vi "AP2_PDS_aquisition.vi"() -> ()   [LabVIEW 2023]
panel:
  in  "Frequency Doubling":bool
  out "RT PDS":cluster{dbl[], i32[]}(graph)
  in  "Cancel Scan Button":bool
  out "FPS":dbl
  in  "Frame timeout (ms)":u32
  in  "Number of buffers":u32
  in  "Region of interest":i32[](array[numeric])
  in  "Stop":bool
  in  "Aquistion Frame Number":i32
  in  "Lower Bound":dbl
  in  "Step Size":dbl
  in  "Upper bound":dbl
  in  "Scan button":bool
  # "AP-2 PDS Acquisition"
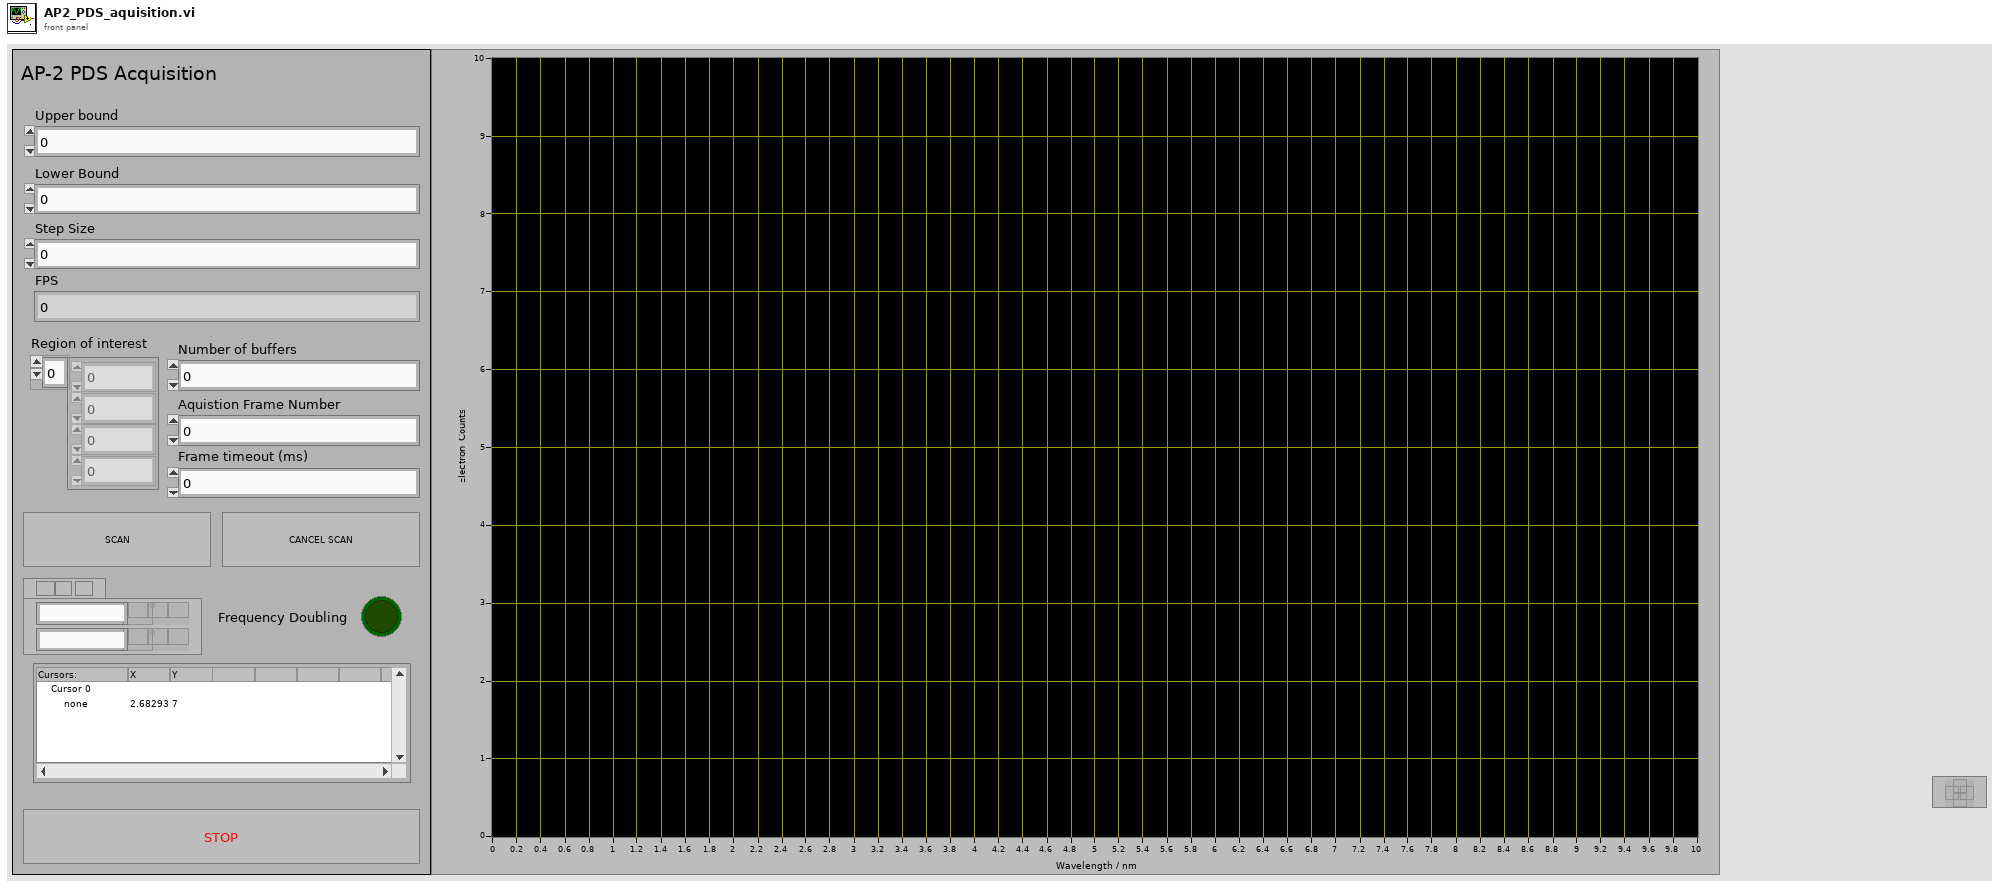
[diagram p1: front panel]
types:
  T1 = cluster{"Region of interest":i32[], "Number of buffers":u32, "Frame timeout (ms)":u32}
  T2 = cluster{"queue out":refnum<queue>, "error out":errorcluster}
  T3 = cluster{"Upper bound":dbl, "Step Size":dbl, "Lower Bound":dbl}
  T4 = cluster{"notifier out":refnum<notifier>, "error out":errorcluster}
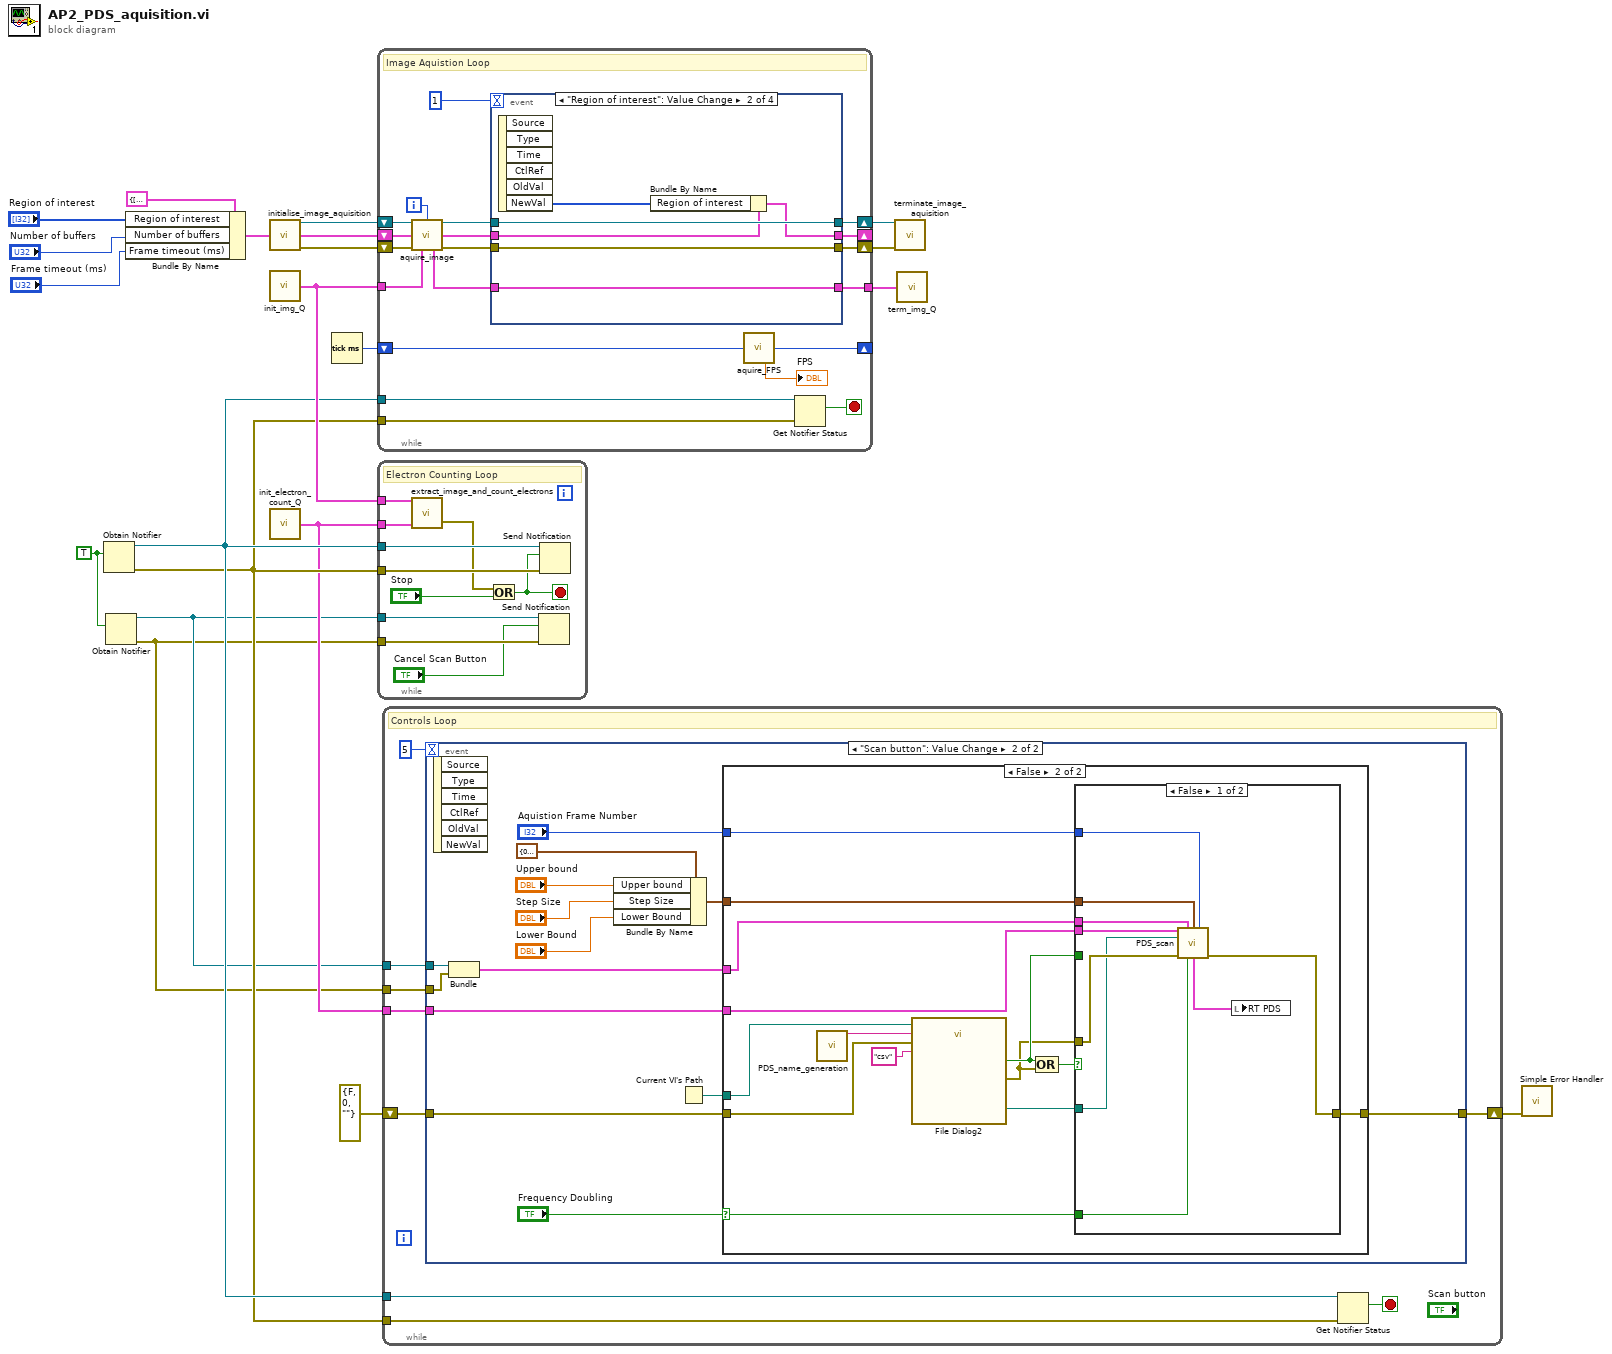
[diagram p0: block diagram]
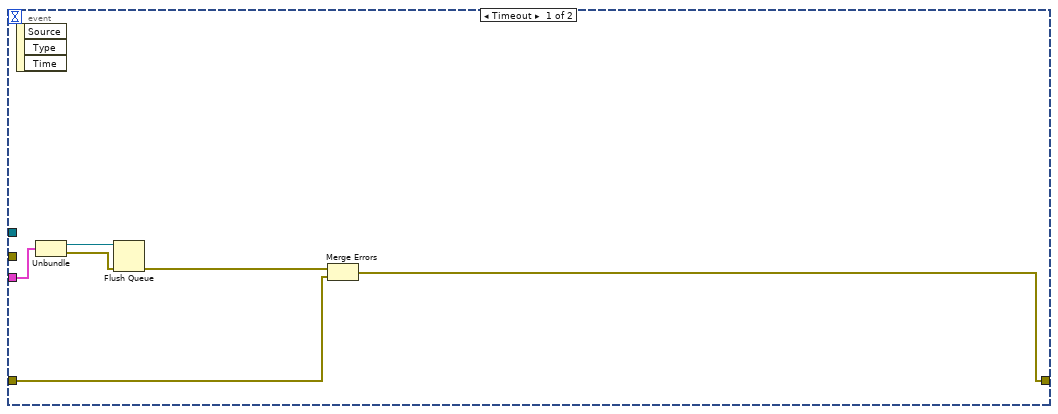
[diagram p2: hidden frame]
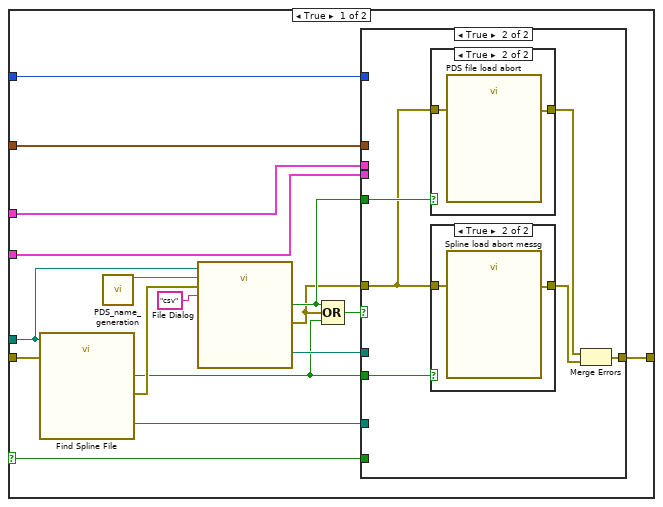
[diagram p3: hidden frame]
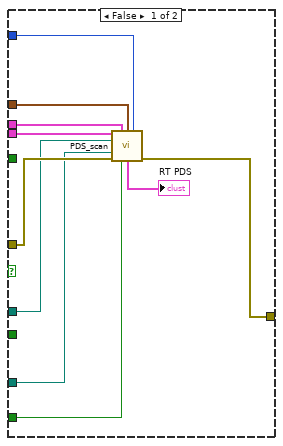
[diagram p4: hidden frame]
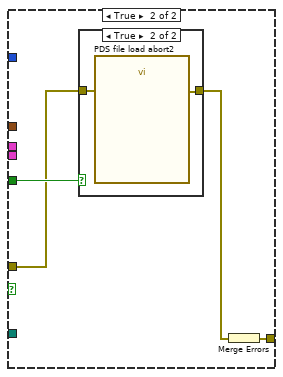
[diagram p7: hidden frame]
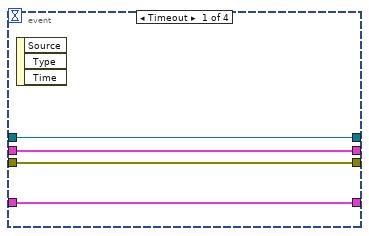
[diagram p9: hidden frame]
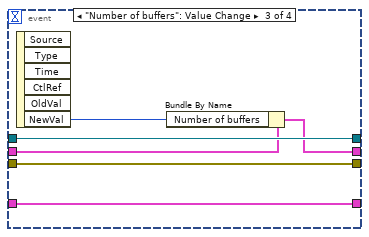
[diagram p10: hidden frame]
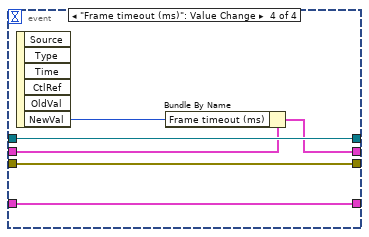
[diagram p11: hidden frame]
diagram:
  w3 = TRUE
  n1 = Obtain Notifier(notification data type=w3) -> (notifier out=w11:refnum<notifier>, error out=w7:errorcluster)  [unwired: 3 in, 1 out]
  n2 = Obtain Notifier(notification data type=w3) -> (notifier out=w2:refnum<notifier>, error out=w1:errorcluster)  [unwired: 3 in, 1 out]
  n3 = Bundle By Name(cluster=T1 {"Region of interest"=[], "Number of buffers"=0, "Frame timeout (ms)"=1000}, "Region of interest"="Region of interest", "Number of buffers"="Number of buffers", "Frame timeout (ms)"="Frame timeout (ms)") -> (w18:T1)
  n4 = call "initialise_image_aquisition.vi"("Imaging Variables In"=w18) -> ("IMAQ Session Out"=w21:refnum<k11>, "Imaging Variables Out"=w17:T1, "error out"=w20:errorcluster)  [unwired: 11 in, 1 out]
  n5 = call "init_img_Q.vi"() -> ("Image Q Out"=w12:T2)  [unwired: 15 in]
  n6 = call "init_electron_count_Q.vi"() -> ("Electron Count Q Out"=w4:T2)  [unwired: 15 in]
  n7 = Tick Count (ms)() -> (millisecond timer value=w13:u32)
  n8 = while {
    shift-right: [w40] -> w15
    shift-left: w21 -> [w37]
    shift-right: [w38] -> w14
    shift-left: w20 -> [w36]
    tunnel: w12 -> [w29]
    tunnel: [w28] -> w16
    shift-right: [w39] -> _
    shift-left: w17 -> [w32]
    shift-right: [w26] -> _
    shift-left: w13 -> [w27]
    tunnel: w11 -> [w25]
    tunnel: w7 -> [w24]
    i -> [w35]
    stop <- w23 stop-if-true
    # "Image Aquistion Loop"
    n9 = call "aquire_image.vi"("IMAQ Session In"=w37, "Buffer to extract"=w35, "Imaging Variables In"=w32, "error in (no error)"=w36, "Img Q Data In"=w29) -> ("IMAQ Session Out"=w34:refnum<k11>, "Imaging Variables Out"=w31:T1, "Img Q Data Out"=w30:T2, "error out"=w33:errorcluster)  [unwired: 7 in]
    n10 = event shown="[1] \"Region of interest\": Value Change" {
      selector: _ -> [_ _ _ _]
      dyn-events: _ -> [_ _ _ _]
      timeout: 1 -> [_ _ _ _]
      tunnel: w34 -> [w45 w51 w57 w63]
      tunnel: w33 -> [w44 w50 w56 w62]
      tunnel: [w45 w51 w57 w63] -> w40
      tunnel: [w44 w50 w56 w62] -> w38
      tunnel: w31 -> [w43 w48 w54 w60]
      tunnel: [w43 w47 w53 w59] -> w39
      tunnel: w30 -> [w42 w49 w55 w61]
      tunnel: [w42 w49 w55 w61] -> w28
      event Timeout {
        n11 = event-data() -> ()  [unwired: 1 in, 3 out]
      }
      event "Region of interest": Value Change {
        n12 = event-data() -> ("NewVal"=w46:i32[])  [unwired: 1 in, 5 out]
        n13 = Bundle By Name(cluster=w48, "Region of interest"=w46) -> (w47:T1)
      }
      event "Number of buffers": Value Change {
        n14 = event-data() -> ("NewVal"=w52:u32)  [unwired: 1 in, 5 out]
        n15 = Bundle By Name(cluster=w54, "Number of buffers"=w52) -> (w53:T1)
      }
      event "Frame timeout (ms)": Value Change {
        n16 = event-data() -> ("NewVal"=w58:u32)  [unwired: 1 in, 5 out]
        n17 = Bundle By Name(cluster=w60, "Frame timeout (ms)"=w58) -> (w59:T1)
      }
    }
    n18 = call "aquire_FPS.vi"("Time Value In /ms"=w27) -> ("Time Value Out /ms"=w26:u32, "FPS"=→"FPS":dbl)  [unwired: 12 in, 1 out]
    n19 = Get Notifier Status(notifier=w25, error in (no error)=w24) -> (current notification=w23:bool)  [unwired: 4 out]
  }
  n20 = while {
    tunnel: w12 -> [w71]
    tunnel: w4 -> [w70]
    tunnel: w11 -> [w73]
    tunnel: w7 -> [w72]
    tunnel: w2 -> [w66]
    tunnel: w1 -> [w65]
    stop <- w67 stop-if-true
    # "Electron Counting Loop"
    n21 = call "extract_image_and_count_electrons.vi"("Image Q In"=w71, "Electron Count Q In"=w70) -> ("error out"=w69:errorcluster)  [unwired: 11 in, 2 out]
    n22 = Or(x=w69, y="Stop") -> (x .or. y?=w67:bool)
    n23 = Send Notification(notification="Cancel Scan Button", notifier=w66, error in (no error)=w65) -> ()  [unwired: 2 out]
    n24 = Send Notification(notification=w67, notifier=w73, error in (no error)=w72) -> ()  [unwired: 2 out]
  }
  n25 = while {
    tunnel: w11 -> [w81]
    tunnel: w7 -> [w80]
    shift-right: [w77] -> w5
    shift-left: errorcluster {"status"=FALSE, "code"=0, "source"=""} ("error out") -> [w78]
    tunnel: w4 -> [w76]
    tunnel: w2 -> [w75]
    tunnel: w1 -> [w74]
    stop <- w79 stop-if-true
    # "Controls Loop"
    n26 = event shown="[1] \"Scan button\": Value Change" {
      selector: _ -> [_ _]
      dyn-events: _ -> [_ _]
      timeout: 5 -> [_ _]
      tunnel: w78 -> [w84 w94]
      tunnel: [w83 w93] -> w77
      tunnel: w76 -> [w87 w92]
      tunnel: w75 -> [_ w91]
      tunnel: w74 -> [_ w90]
      event Timeout {
        n27 = event-data() -> ()  [unwired: 1 in, 3 out]
        n28 = Unbundle(w87) -> ("queue out"=w86:refnum<queue>, "error out"=w85:errorcluster)
        n29 = Flush Queue(queue=w86, error in (no error)=w85) -> (error out=w88:errorcluster)  [unwired: 2 out]
        n30 = Merge Errors(w88, w84) -> (w83:errorcluster)
      }
      event "Scan button": Value Change {
        n31 = event-data() -> ()  [unwired: 1 in, 6 out]
        n32 = Bundle("notifier out"=w91, "error out"=w90) -> (w89:T4)  [unwired: 1 in]
        n33 = Bundle By Name(cluster=T3 {"Upper bound"=0.0, "Step Size"=0.0, "Lower Bound"=0.0}, "Upper bound"="Upper bound", "Step Size"="Step Size", "Lower Bound"="Lower Bound") -> (w97:T3)
        n34 = Current VI's Path() -> (path=w95:path)
        n35 = case shown="False" "Frequency Doubling" {
          selector: "Frequency Doubling" -> [w104 w144]
          tunnel: w97 -> [w107 w147]
          tunnel: "Aquistion Frame Number" -> [w106 w146]
          tunnel: w95 -> [w115 w153]
          tunnel: w94 -> [w119 w143]
          tunnel: [w108 w148] -> w93
          tunnel: w92 -> [w105 w145]
          tunnel: w89 -> [w103 w142]
          frame True {
            n36 = call "Find Spline File"("start path"=w115, "error in"=w119) -> ("selected path"=w112:path, "cancelled"=w111:bool, "error out"=w116:errorcluster)  [unwired: 10 in, 1 out]
            n37 = call "PDS_name_generation.vi"() -> ("Generic Name"=w118:string)  [unwired: 15 in]
            n38 = call "File Dialog"("start path"=w115, "default name"=w118, "error in"=w116, "pattern (all files)"="csv") -> ("selected path"=w113:path, "cancelled"=w110:bool, "error out"=w109:errorcluster)  [unwired: 8 in, 1 out]
            n39 = Compound Arithmetic op=OR(w110, w109, w111) -> (w114:bool)
            n40 = case shown="True" w114 {
              tunnel: w113 -> [w122 _]
              tunnel: w112 -> [w121 _]
              tunnel: w111 -> [_ w135]
              tunnel: w109 -> [w125 w133]
              tunnel: w110 -> [_ w134]
              tunnel: [w124 w131] -> w108
              tunnel: w107 -> [w127 _]
              tunnel: w106 -> [w126 _]
              tunnel: w105 -> [w129 _]
              tunnel: w104 -> [w123 _]
              tunnel: w103 -> [w120 _]
              frame False {
                n41 = call "PDS_scan.vi"("Electron Count Q In"=w129, "Cancel scan notifier"=w120, "Scan Range Data"=w127, "Aquistion Frame Number"=w126, "file path (dialog if empty)"=w122, "Tuning Spline Path"=w121, "error in (no error)"=w125, "Doubled?"=w123) -> ("RT PDS"=→"RT PDS":cluster{dbl[], i32[]}, "error out"=w124:errorcluster)  [unwired: 6 in]
              }
              frame True {
                n42 = case shown="True" w134 {
                  tunnel: w133 -> [w136 w138]
                  tunnel: [w136 w137] -> w132
                  frame False {
                  }
                  frame True {
                    n43 = call "PDS file load abort"("error in (no error)"=w138) -> ("error out"=w137:errorcluster)  [unwired: 9 in, 1 out]
                  }
                }
                n44 = case shown="True" w135 {
                  tunnel: w133 -> [w139 w141]
                  tunnel: [w139 w140] -> w130
                  frame False {
                  }
                  frame True {
                    n45 = call "Spline load abort messg"("error in (no error)"=w141) -> ("error out"=w140:errorcluster)  [unwired: 9 in, 1 out]
                  }
                }
                n46 = Merge Errors(w132, w130) -> (w131:errorcluster)
              }
            }
          }
          frame False {
            n47 = call "PDS_name_generation.vi"() -> ("Generic Name"=w155:string)  [unwired: 15 in]
            n48 = call "File Dialog2"("start path"=w153, "default name"=w155, "error in"=w143, "pattern (all files)"="csv") -> ("selected path"=w151:path, "cancelled"=w150:bool, "error out"=w149:errorcluster)  [unwired: 8 in, 1 out]
            n49 = Compound Arithmetic op=OR(w150, w149) -> (w152:bool)
            n50 = case shown="False" w152 {
              tunnel: w151 -> [w158 _]
              tunnel: w149 -> [w161 w167]
              tunnel: w150 -> [_ w168]
              tunnel: [w160 w165] -> w148
              tunnel: w147 -> [w163 _]
              tunnel: w146 -> [w162 _]
              tunnel: w145 -> [w164 _]
              tunnel: w144 -> [w159 _]
              tunnel: w142 -> [w157 _]
              frame False {
                n51 = call "PDS_scan.vi"("Electron Count Q In"=w164, "Cancel scan notifier"=w157, "Scan Range Data"=w163, "Aquistion Frame Number"=w162, "file path (dialog if empty)"=w158, "error in (no error)"=w161, "Doubled?"=w159) -> ("RT PDS"=w156:cluster{dbl[], i32[]}, "error out"=w160:errorcluster)  [unwired: 7 in]
                n52 = local write "RT PDS"(w156) -> ()
              }
              frame True {
                n53 = case shown="True" w168 {
                  tunnel: w167 -> [w169 w171]
                  tunnel: [w169 w170] -> w166
                  frame False {
                  }
                  frame True {
                    n54 = call "PDS file load abort2"("error in (no error)"=w171) -> ("error out"=w170:errorcluster)  [unwired: 9 in, 1 out]
                  }
                }
                n55 = Merge Errors(w166) -> (w165:errorcluster)
              }
            }
          }
        }
      }
    }
    n56 = Get Notifier Status(notifier=w81, error in (no error)=w80) -> (current notification=w79:bool)  [unwired: 4 out]
  }
  n57 = call "terminate_image_aquisition.vi"("IMAQ Session In"=w15, "error in (no error)"=w14) -> ()  [unwired: 13 in, 1 out]
  n58 = call "term_img_Q.vi"("Image Q Out"=w16) -> ()  [unwired: 14 in, 1 out]
  n59 = call <vilib>:"Simple Error Handler.vi"("error in (no error)"=w5) -> ()  [unwired: 4 in, 5 out]
